vi "Write Deadband.vi"(8 "error in (no error)":cluster{"状态":bool, "代码":i32, "源":string} caption="错误输入（无错误）", 10 "死区":T1, 11 "水位控制器输入":refnum<class "Level Controller.lvclass">) -> (0 "error out":cluster{"状态":bool, "代码":i32, "源":string} caption="错误输出", 3 "水位控制器输出":refnum<class "Level Controller.lvclass">)   [LabVIEW 2015, in "Level Controller.lvlib" / "Level Controller.lvclass"]
doc: "写入水位控制器的死区范围。高点和低点可以设为同一个值，但如低点的值大于高点的值，该方法将返回错误代码1。"
uses:
  Level Controller.lvclass
  Deadband.ctl
  Level Controller.lvclass/Level Controller.ctl
  <vilib>/Utility/error.llb/Error Cluster From Error Code.vi
  <vilib>/ErrorRing/Error Ring.xnode
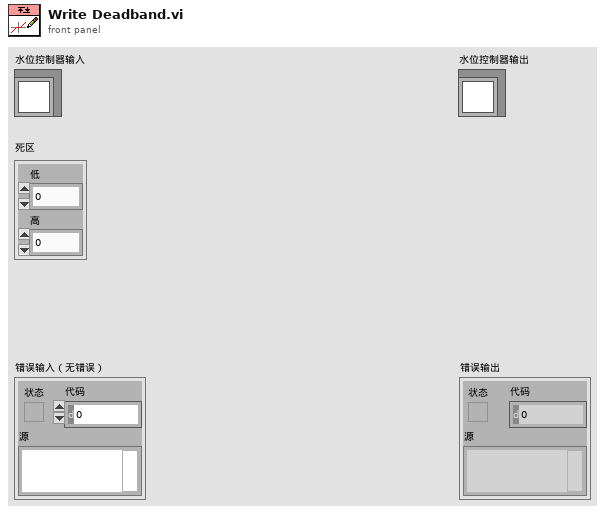
[diagram p1: front panel]
types:
  T1 = typedef "Level Controller.lvlib/Level Controller.lvclass/Deadband.ctl" = cluster{"低":dbl, "高":dbl}
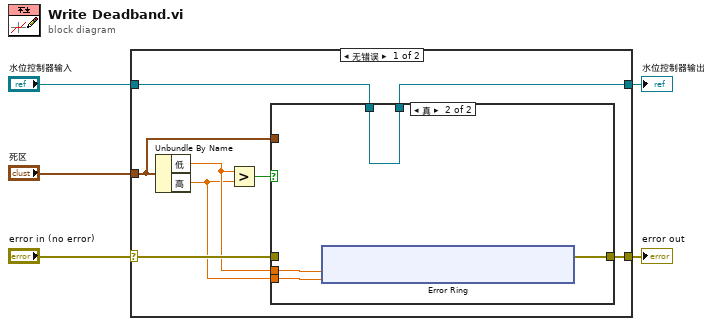
[diagram p0: block diagram]
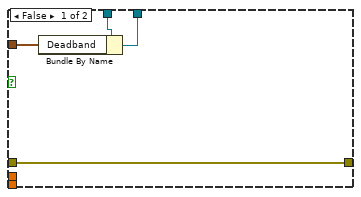
[diagram p2: hidden frame]
diagram:
  n1 = case shown="无错误" "error in (no error)" {
    selector: "error in (no error)" -> [w8 w30]
    tunnel: [w9 w30] -> w4
    tunnel: [w12 w31] -> w2
    tunnel: "水位控制器输入" -> [w13 w31]
    tunnel: "死区" -> [w10 _]
    frame No Error {
      n2 = Unbundle By Name(w10) -> ("低"=w7:dbl, "高"=w6:dbl)
      n3 = Greater?(x=w7, y=w6) -> (0:w11:bool)
      n4 = case shown="真" w11 {
        tunnel: w13 -> [w17 w21]
        tunnel: [w16 w21] -> w12
        tunnel: w10 -> [w15 _]
        tunnel: [w14 w20] -> w9
        tunnel: w8 -> [w14 _]
        tunnel: w7 -> [_ w19]
        tunnel: w6 -> [_ w18]
        frame False {
          n5 = Bundle By Name(cluster=w17, "Deadband"=w15) -> (w16:refnum<class "Level Controller.lvclass">)
        }
        frame True {
          n6 = xnode "Error Ring"("参数 0"=w19, "参数 1"=w18) -> ("错误输出"=w20:errorcluster)
        }
      }
    }
    frame Error {
    }
  }
  "error out" <- w4
  "水位控制器输出" <- w2
